vi "Get Server DLL Path.vi"() -> (0 "Server dll path":path)   [LabVIEW 2020, in "grpc-lvsupport-release.lvlib"]
uses:
  <vilib>/gRPC/LabVIEW gRPC Library/grpc-lvsupport-release.lvlib
  <vilib>/Utility/LVLibp/NI_PackedLibraryUtility.lvlib
  <vilib>/Utility/sysdir.llb/System Directory Type.ctl
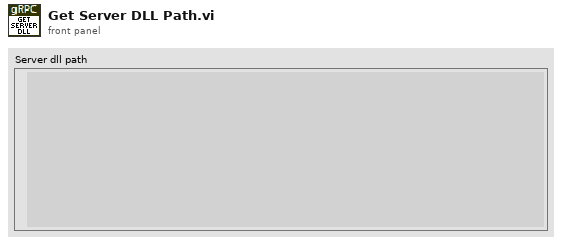
[diagram p1: front panel]
types:
  T1 = typedef "System Directory Type.ctl" = i32
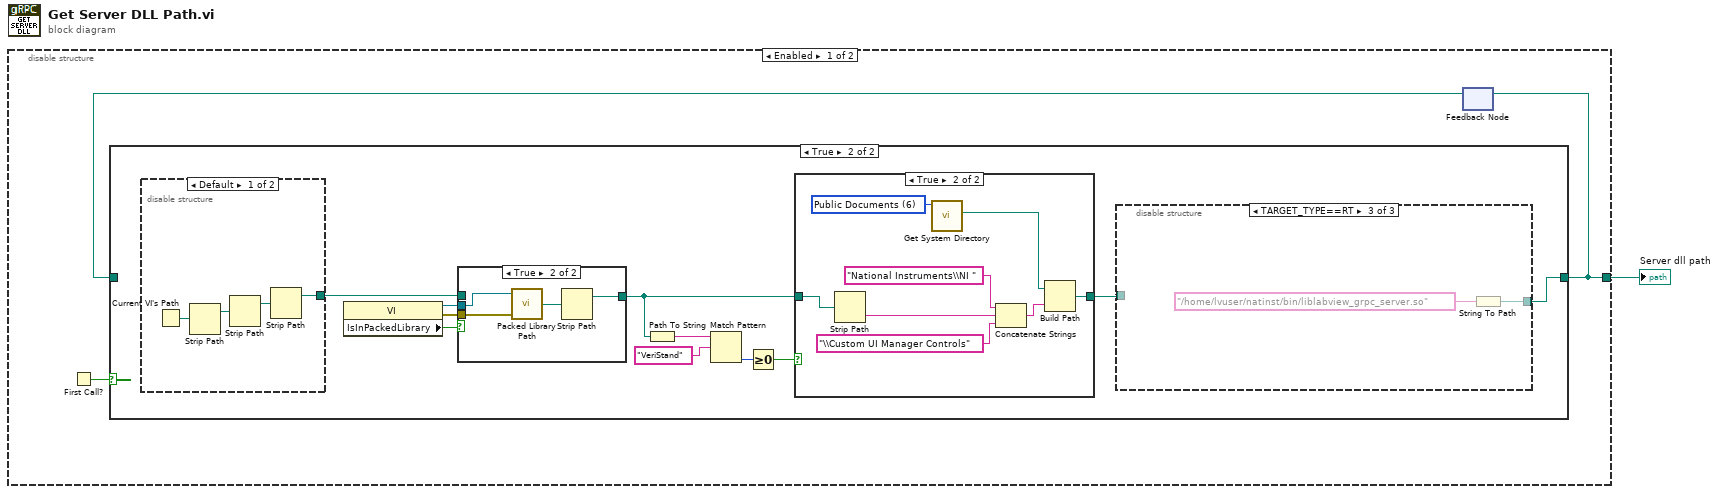
[diagram p0: block diagram]
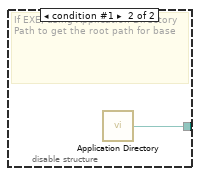
[diagram p5: hidden frame]
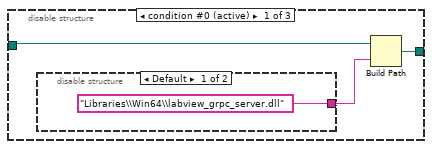
[diagram p6: hidden frame]
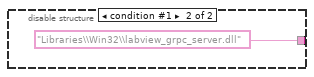
[diagram p7: hidden frame]
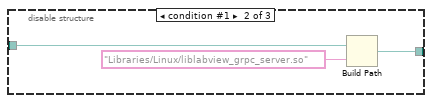
[diagram p8: hidden frame]
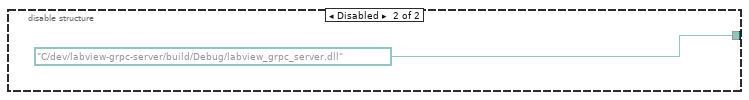
[diagram p9: hidden frame]
diagram:
  n1 = disable-structure shown="Enabled" {
    disable-tunnel: [w3 path "C:/dev/labview-grpc-server/build/Debug/labview_grpc_server.dll" ("Server dll path")] -> w1
    frame Enabled {
      n2 = First Call?() -> (First Call?: T/F=w4:bool)
      n3 = feedback #1() -> (w2:path)  [unwired: 1 in]
      n4 = case shown="True" w4 {
        tunnel: [w5 w16] -> w3
        tunnel: w2 -> [w5 _]
        frame False {
        }
        frame True {
          n5 = disable-structure shown="Default" {
            disable-tunnel: [w31 w35] -> w12
            frame condition #0 (active) {
              n6 = Current VI's Path() -> (path=w33:path)
              n7 = Strip Path(path=w33) -> (stripped path=w34:path)  [unwired: 1 out]
              n8 = Strip Path(path=w34) -> (stripped path=w32:path)  [unwired: 1 out]
              n9 = Strip Path(path=w32) -> (stripped path=w31:path)  [unwired: 1 out]
            }
            frame condition #1 {
              # "If EXE, using Application Directory Path to get the root path for base"
              n10 = call <vilib>:"Application Directory.vi"() -> ("Application Directory"=w35:path)
            }
          }
          n11 = property class="VI"() -> (reference out=w14:refnum<vi>, error out=w15:errorcluster, "IsInPackedLibrary"=w13:bool)  [unwired: 2 in]
          n12 = case shown="True" w13 {
            tunnel: w14 -> [_ w30]
            tunnel: w15 -> [_ w29]
            tunnel: [w26 w28] -> w7
            tunnel: w12 -> [w26 _]
            frame False {
            }
            frame True {
              n13 = call <vilib>:"Packed Library Path.vi"("error in (no error)"=w29, "vi reference"=w30) -> ("packed library path"=w27:path)  [unwired: 1 in, 2 out]
              n14 = Strip Path(path=w27) -> (stripped path=w28:path)  [unwired: 1 out]
            }
          }
          n15 = Path To String(path=w7) -> (string=w11:string)
          n16 = Match Pattern(string=w11, regular expression="VeriStand") -> (offset past match=w9:i32)  [unwired: 1 in, 3 out]
          n17 = Greater Or Equal To 0?(x=w9) -> (x >= 0?=w8:bool)
          n18 = case shown="True" w8 {
            tunnel: w7 -> [w17 w24]
            tunnel: [w17 w18] -> w6
            frame False {
            }
            frame True {
              w25 = T1 6 items=["User Home"=0, "User Desktop"=1, "User Documents"=2, "User Application Data"=3, "User Preferences"=4, "User Temporary"=5, "Public Documents"=6, "Public Application Data"=7, "Public Preferences"=8, "Public Cache"=13, "System Core Libraries"=9, "System Installed Libraries"=10, "Application Files"=11, "Boot Volume Root"=12] ("system directory type")
              n19 = Strip Path(path=w24) -> (name=w21:string)  [unwired: 1 out]
              n20 = call <vilib>:"Get System Directory.vi"("system directory type"=w25) -> ("system directory"=w23:path)  [unwired: 10 in]
              n21 = Concatenate Strings("National Instruments\\NI " ("regular expression"), w21, "\\Custom UI Manager Controls" ("regular expression")) -> (w19:string)
              n22 = Build Path(base path=w23, name or relative path=w19) -> (appended path=w18:path)
            }
          }
          n23 = disable-structure shown="TARGET_TYPE==RT" {
            disable-tunnel: w6 -> [w36 w43 _]
            disable-tunnel: [w37 w42 w44] -> w16
            frame condition #0 (active) {
              n24 = disable-structure shown="Default" {
                disable-tunnel: ["Libraries\\Win64\\labview_grpc_server.dll" ("name or relative path") "Libraries\\Win32\\labview_grpc_server.dll" ("name or relative path")] -> w38
                frame condition #0 (active) {
                }
                frame condition #1 {
                }
              }
              n25 = Build Path(base path=w36, name or relative path=w38) -> (appended path=w37:path)
            }
            frame condition #1 {
              n26 = Build Path(base path=w43, name or relative path="Libraries/Linux/liblabview_grpc_server.so") -> (appended path=w42:path)
            }
            frame condition #2 {
              n27 = String To Path(string="/home/lvuser/natinst/bin/liblabview_grpc_server.so" ("name or relative path")) -> (path=w44:path)
            }
          }
        }
      }
      n28 = feedback-in #1(w3) -> ()
    }
    frame Disabled {
    }
  }
  "Server dll path" <- w1
